vi "PRL DW Clean Data CSG 2D.vi"(7 "Remove Bad Data?":bool, 11 "Array In":csg[][](array[numeric])) -> (1 "Bad Data Ratio":dbl, 2 "Bad Data?":bool, 3 "Array Out":csg[][](array[numeric]))   [LabVIEW 2013, in "PMU Recorder Light.lvlib"]
uses:
  PMU Recorder Light.lvlib
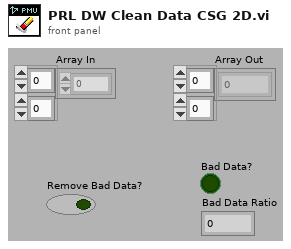
[diagram p1: front panel]
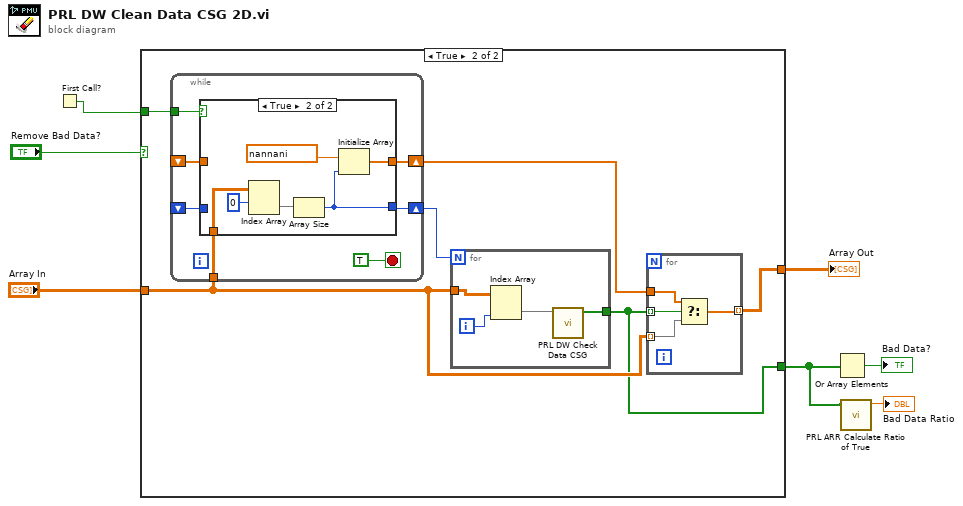
[diagram p0: block diagram]
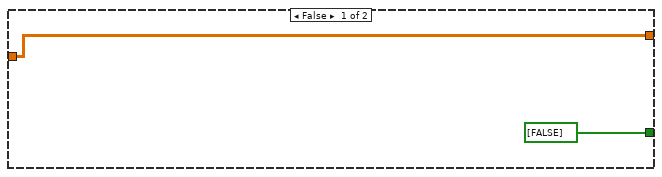
[diagram p2: hidden frame]
diagram:
  n1 = First Call?() -> (First Call?: T/F=w3:bool)
  n2 = case shown="True" "Remove Bad Data?" {
    tunnel: [w9 w11] -> w7
    tunnel: [bool[] [FALSE] w10] -> w1
    tunnel: "Array In" -> [w9 w13]
    tunnel: w3 -> [_ w14]
    frame False {
    }
    frame True {
      n3 = while {
        tunnel: w13 -> [w26]
        tunnel: w14 -> [w24]
        shift-right: [w22] -> w12
        shift-left: _ -> [w20]
        shift-right: [w25] -> w15
        shift-left: _ -> [w21]
        stop <- TRUE stop-if-true
        n4 = case shown="True" w24 {
          tunnel: w26 -> [_ w34]
          tunnel: [w27 w31] -> w25
          tunnel: [w28 w29] -> w22
          tunnel: w21 -> [w27 _]
          tunnel: w20 -> [w28 _]
          frame False {
          }
          frame True {
            n5 = Index Array(array=w34, index (row)=0) -> (element=w32:csg[])  [unwired: 1 in]
            n6 = Array Size(array=w32) -> (size(s)=w31:i32)
            n7 = Initialize Array(csg nan+nani ("element"), w31) -> (w29:csg[])
          }
        }
      }
      n8 = for {
        N: w15 -> [_]
        tunnel: w13 -> [w38]
        tunnel: [w35] -> w10
        i -> [w37]
        n9 = Index Array(array=w38, index (col)=w37) -> (element=w36:csg[])  [unwired: 1 in]
        n10 = call "PRL DW Check Data CSG.vi"("Data"=w36) -> ("Bad Data?"=w35:bool[])  [unwired: 10 in]
      }
      n11 = for {
        tunnel: w10 -> [w19] mode=indexing
        tunnel: w13 -> [w17] mode=indexing
        tunnel: w12 -> [w18]
        tunnel: [w16] -> w11 mode=indexing
        n12 = Select(t=w18, s=w19, f=w17) -> (s? t:f=w16:csg[])
      }
    }
  }
  "Array Out" <- w7
  n13 = Or Array Elements(Boolean array=w1) -> (logical OR=→"Bad Data?":bool)
  n14 = call "PRL ARR Calculate Ratio of True.vi"("Array"=w1) -> ("True Ratio"=→"Bad Data Ratio":dbl)  [unwired: 10 in]
